vi "Control Lamp.vi"(4 "Alarm State":bool, 6 "Lamp State":bool, 8 "error in (no error)":errorcluster, 10 "Function Choose":T1(ring), 11 "VISA resource name":refnum<visa-resource-name>) -> (0 "error out":errorcluster, 3 "VISA resource name out":refnum<visa-resource-name>)   [LabVIEW 2020]
uses:
  201833fa-8973-4c29-a2c9-f1b8bd81a6a5.vi
  <vilib>/Instr/_visa.llb/VISA Configure Serial Port (Instr).vi
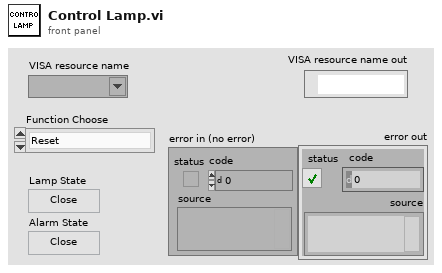
[diagram p1: front panel]
types:
  T1 = enum16{"Reset", "Yellow Lamp&Alarm", "Green Lamp&Alarm", "Red Lamp&Alarm"}
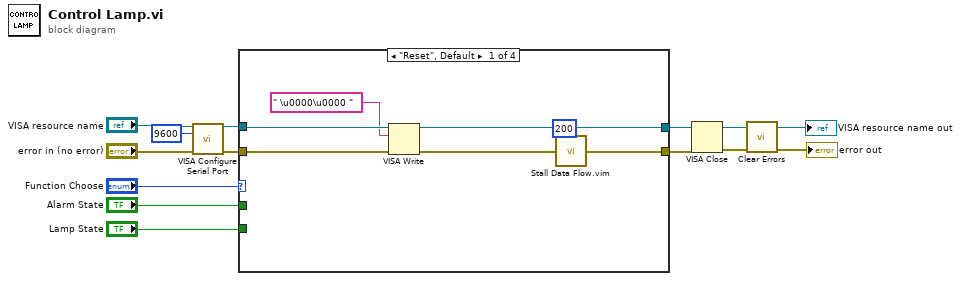
[diagram p0: block diagram]
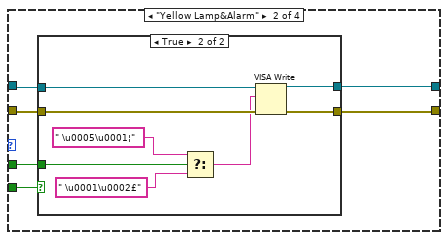
[diagram p2: hidden frame]
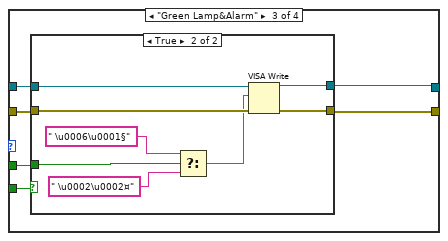
[diagram p4: hidden frame]
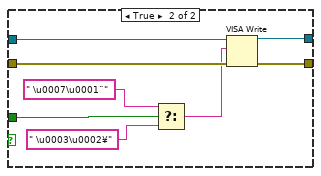
[diagram p7: hidden frame]
diagram:
  n1 = call-poly "VISA Configure Serial Port"("VISA resource name"="VISA resource name", "baud rate (9600)"=u32 9600, "error in (no error)"="error in (no error)") -> ("VISA resource name out"=w5:refnum<visa-resource-name>, "error out"=w9:errorcluster)  [unwired: 11 in]
  n2 = case shown="\"Reset\", Default" "Function Choose" {
    tunnel: "Lamp State" -> [_ w21 w38 w54]
    tunnel: "Alarm State" -> [_ w20 w39 w55]
    tunnel: w9 -> [w19 w24 w40 w56]
    tunnel: w5 -> [w18 w25 w41 w57]
    tunnel: [w17 w22 w37 w53] -> w3
    tunnel: [w14 w23 w36 w52] -> w4
    frame "Reset", Default {
      n3 = VISA Write(VISA resource name=w18, write buffer=" \u0000\u0000 ", error in (no error)=w19) -> (VISA resource name out=w17:refnum<visa-resource-name>, error out=w16:errorcluster)  [unwired: 1 out]
      n4 = call "Stall Data Flow.vim"("value in"=w16, "milliseconds to wait"=u32 200) -> ("value out"=w14:errorcluster)  [unwired: 1 out]
    }
    frame "Yellow Lamp&Alarm" {
      n5 = case shown="True" w21 {
        tunnel: w25 -> [w27 w35]
        tunnel: w24 -> [w26 w34]
        tunnel: [w26 w33] -> w23
        tunnel: [w27 w32] -> w22
        tunnel: w20 -> [_ w31]
        frame False {
        }
        frame True {
          n6 = Select(t=" \u0005\u0001¦" ("write buffer"), s=w31, f=" \u0001\u0002£" ("write buffer")) -> (s? t:f=w28:string)
          n7 = VISA Write(VISA resource name=w35, write buffer=w28, error in (no error)=w34) -> (VISA resource name out=w32:refnum<visa-resource-name>, error out=w33:errorcluster)  [unwired: 1 out]
        }
      }
    }
    frame "Green Lamp&Alarm" {
      n8 = case shown="True" w38 {
        tunnel: w41 -> [w43 w51]
        tunnel: w40 -> [w42 w50]
        tunnel: [w42 w49] -> w36
        tunnel: [w43 w48] -> w37
        tunnel: w39 -> [_ w47]
        frame False {
        }
        frame True {
          n9 = Select(t=" \u0006\u0001§" ("write buffer"), s=w47, f=" \u0002\u0002¤" ("write buffer")) -> (s? t:f=w44:string)
          n10 = VISA Write(VISA resource name=w51, write buffer=w44, error in (no error)=w50) -> (VISA resource name out=w48:refnum<visa-resource-name>, error out=w49:errorcluster)  [unwired: 1 out]
        }
      }
    }
    frame "Red Lamp&Alarm" {
      n11 = case shown="False" w54 {
        tunnel: w57 -> [w59 w67]
        tunnel: w56 -> [w58 w66]
        tunnel: [w58 w65] -> w52
        tunnel: [w59 w64] -> w53
        tunnel: w55 -> [_ w63]
        frame False {
        }
        frame True {
          n12 = Select(t=" \u0007\u0001¨" ("write buffer"), s=w63, f=" \u0003\u0002¥" ("write buffer")) -> (s? t:f=w60:string)
          n13 = VISA Write(VISA resource name=w67, write buffer=w60, error in (no error)=w66) -> (VISA resource name out=w64:refnum<visa-resource-name>, error out=w65:errorcluster)  [unwired: 1 out]
        }
      }
    }
  }
  "VISA resource name out" <- w3
  n14 = VISA Close(VISA resource name=w3, error in (no error)=w4) -> (error out=w2:errorcluster)
  n15 = call <vilib>:"Clear Errors.vi"("error in (no error)"=w2) -> ("error out"=→"error out":errorcluster)  [unwired: 5 in, 1 out]
